vi "ex_GetSystemDecimalSeparator.vi"() -> (2 "Decimal Seperator":string)   [LabVIEW 2017]
panel:
  out "resulting string":string="0,000000"
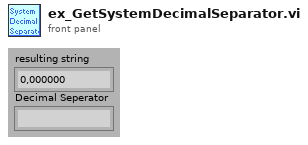
[diagram p1: front panel]
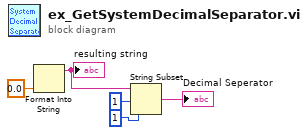
[diagram p0: block diagram]
diagram:
  n1 = Format Into String(0.0 ("input 1")) -> (resulting string=w4:string)  [unwired: 3 in, 1 out]
  "resulting string" <- w4
  n2 = String Subset(string=w4, offset (0)=1, length (rest)=1 ("length (rest)")) -> (substring=→"Decimal Seperator":string)
